vi "SwitchBoard_error.vi"(8 "error constant":errorcluster, 10 "Source":string, 11 "Code":i32) -> (0 "error IO":errorcluster)   [LabVIEW 2016]
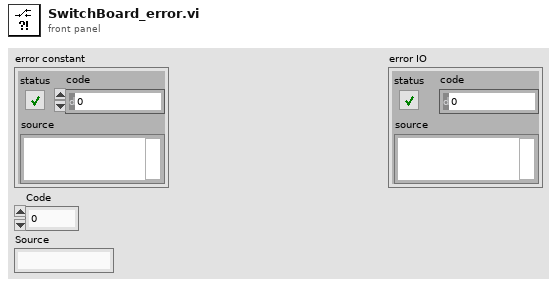
[diagram p1: front panel]
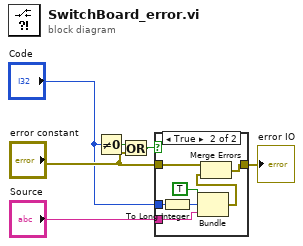
[diagram p0: block diagram]
diagram:
  n1 = Not Equal To 0?(x="Code") -> (x != 0?=w6:bool)
  n2 = Or(x=w6, y="error constant") -> (x .or. y?=w5:bool)
  n3 = case shown="True" w5 {
    tunnel: "error constant" -> [w7 w14]
    tunnel: [w7 w10] -> w3
    tunnel: "Code" -> [_ w9]
    tunnel: "Source" -> [_ w8]
    frame False {
    }
    frame True {
      n4 = To Long Integer(number=w9) -> (32bit integer=w11:i32)
      n5 = Bundle(TRUE, w11, "Source"=w8) -> (w12:cluster{bool, i32, "Source ":string})  [unwired: 1 in]
      n6 = Merge Errors(w14, w12) -> (w10:errorcluster)
    }
  }
  "error IO" <- w3
